vi "901x 9870 DMA Write (Sub).vi"(8 "error in":errorcluster, 10 "Send Data":string, 11 "FPGA In":T1) -> (0 "error out":errorcluster, 1 "Byte Count":u32, 3 "FPGA Out":T1, 4 "Timed Out":bool, 6 "FPGA Error":errorcluster)   [LabVIEW 2012]
uses:
  901x DMA FPGA Reference.ctl
  FPGA Function.ctl
  <vilib>/Utility/error.llb/Error Cluster From Error Code.vi
  <vilib>/rvi/errors/niLvFpgaAdjustHostInterfaceError.vi
  <vilib>/rvi/interface/nirviReadWriteControl/nirviReadWriteControl.xnode
  Program Files (x86)/National Instruments/LabVIEW 2012/examples/CompactRIO/Module Specific/NI 987x/Serial Loopback/FPGA Bitfiles/NI-987xSerialLoo_FPGATarget4_9870InterfaceDMA_lMxNdb7MvEs.lvbitx
  Program Files (x86)/National Instruments/LabVIEW 2012/examples/CompactRIO/Module Specific/NI 987x/Serial Loopback/VIs/9870 Interface DMA (FPGA).vi
  <vilib>/rvi/interface/nirviMethod/nirviMethod.xnode
  <vilib>/rvi/errors/niLvFpgaMergeErrorWithErrorCode.vi
  NiFpgaLv.dll
  <vilib>/FPGAPlugInAG/cRIO-9113/niLvFpga_WriteFifo_cRIO-9113.vi
  <vilib>/FPGAPlugInAG/cRIO-9113/niLvFpga_AcknowledgeIrq_cRIO-9113.vi
  <vilib>/rvi/interface/nirviMethod/StockFPGA_InlinedMethodWaitForSingleIRQ.vi
  <vilib>/FPGAPlugInAG/cRIO-9113/niLvFpga_WaitOnIrq_cRIO-9113.vi
panel:
  # "INPUTS"
  # "OUTPUTS"
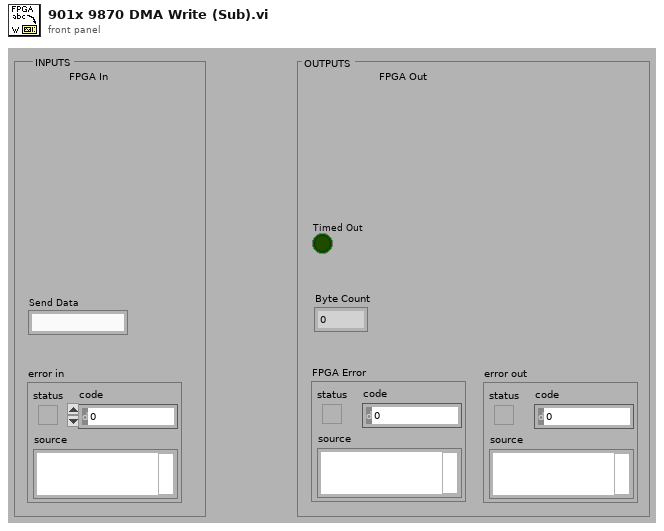
[diagram p1: front panel]
types:
  T1 = typedef "901x DMA FPGA Reference.ctl" = refnum<k20>
  T2 = typedef "FPGA Function.ctl" = enum16{"Do Nothing", "Write", "Read"}
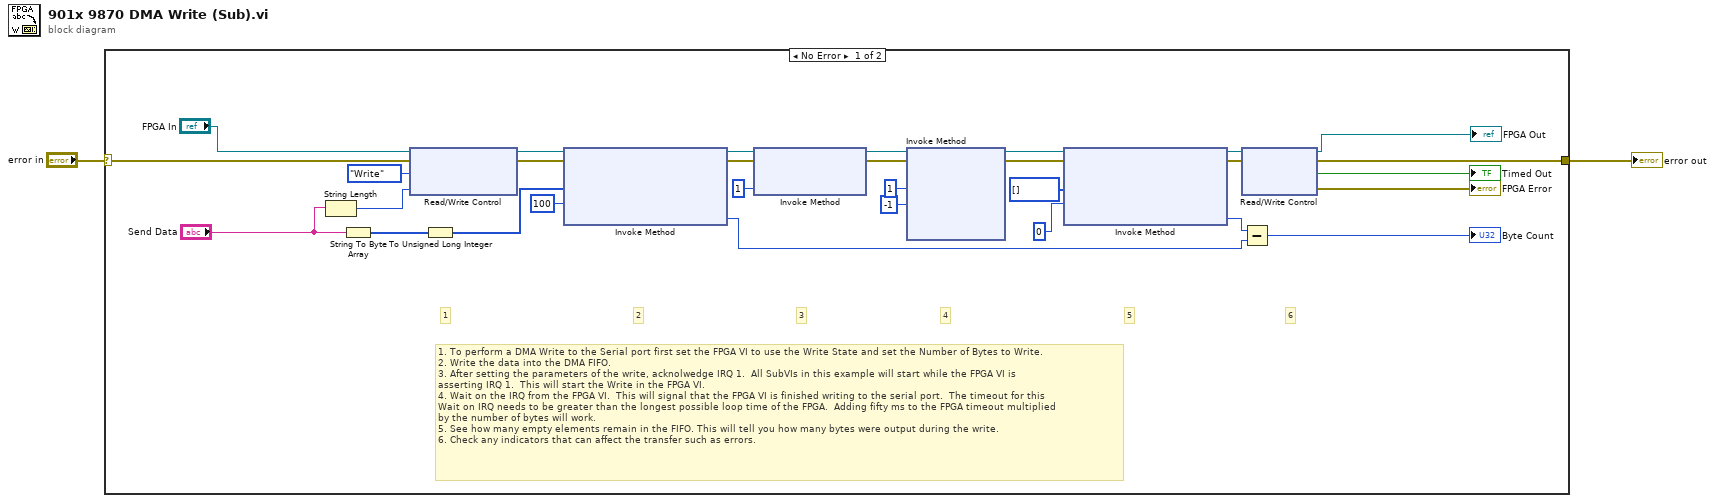
[diagram p0: block diagram]
diagram:
  n1 = case shown="No Error" "error in" {
    selector: "error in" -> [w5 w33]
    tunnel: [w32 w33] -> w2
    frame No Error {
      # "5"
      # "6"
      # "4"
      # "3"
      # "2"
      # "1"
      # "1. To perform a DMA Write to the Serial port first set the FPGA VI to use the Write State and set the Number of Bytes to Write.\n2. Write the data into the DMA FIFO.\n3. After setting the parameters of the write, acknolwedge IRQ 1.  All SubVIs in this example will start while the FPGA VI is \nasserting IRQ 1.  This will start the Write in the FPGA VI.\n4. Wait on the IRQ from the FPGA VI.  This will signal that the FPGA VI is finished writing to the serial port.  The timeout for this \nWait on IRQ needs to be greater than the longest possible loop time of the FPGA.  Adding fifty ms to the FPGA timeout multiplied \nby the number of bytes will work.\n5. See how many empty elements remain in the FIFO. This will tell you how many bytes were output during the write.\n6. Check any indicators that can affect the transfer such as errors."
      n2 = String Length(string="Send Data") -> (length=w4:i32)
      n3 = String To Byte Array(string="Send Data") -> (unsigned byte array=w17:u8[])
      n4 = xnode "Read/Write Control"("FPGA VI Reference In"="FPGA In", "error in"=w5, "Op Control"=FPGA_Function."Write", "Number of Bytes"=w4) -> ("FPGA VI Reference Out"=w30:T1, "error out"=w29:errorcluster)
      n5 = To Unsigned Long Integer(number=w17) -> (unsigned 32bit integer=w16:u32[])
      n6 = xnode "Invoke Method"("FPGA VI Reference In"=w30, "error in"=w29, "Data"=w16, "Timeout (ms)"=100) -> ("FPGA VI Reference Out"=w26:T1, "error out"=w25:errorcluster, "Empty Elements Remaining"=w7:u32)
      n7 = xnode "Invoke Method"("FPGA VI Reference In"=w26, "error in"=w25, "IRQ Number(s)"=1) -> ("FPGA VI Reference Out"=w24:T1, "error out"=w23:errorcluster)
      n8 = xnode "Invoke Method"("FPGA VI Reference In"=w24, "error in"=w23, "IRQ Number(s)"=1, "Timeout (ms)"=-1) -> ("FPGA VI Reference Out"=w14:T1, "error out"=w13:errorcluster)  [unwired: 2 out]
      n9 = xnode "Invoke Method"("FPGA VI Reference In"=w14, "error in"=w13, "Data"=u32[] [], "Timeout (ms)"=0) -> ("FPGA VI Reference Out"=w12:T1, "error out"=w11:errorcluster, "Empty Elements Remaining"=w8:u32)
      n10 = xnode "Read/Write Control"("FPGA VI Reference In"=w12, "error in"=w11) -> ("FPGA VI Reference Out"=→"FPGA Out":T1, "error out"=w32:errorcluster, "Timed Out"=→"Timed Out":bool, "error out"=→"FPGA Error":errorcluster)
      n11 = Subtract(x=w8, y=w7) -> (x-y=→"Byte Count":u32)
    }
    frame Error {
    }
  }
  "error out" <- w2
